vi "ROI 2 Trap Cluster.vi"(5 "Amplitudes":dbl[](array[numeric]), 6 "Switch X/Y":bool, 7 "Group":bool[](array[boolean]), 8 "Trap Cluster in":T2, 9 "Z":dbl[](array[numeric]), 10 "ROI":T1) -> (0 "Group out":bool[](array[boolean]), 1 "Z out":dbl[](array[numeric]), 2 "Amplitudes out":dbl[](array[numeric]), 3 "Trap Cluster Out":T2, 4 "Update display":bool)   [LabVIEW 8.6]
uses:
  Trap cluster.ctl
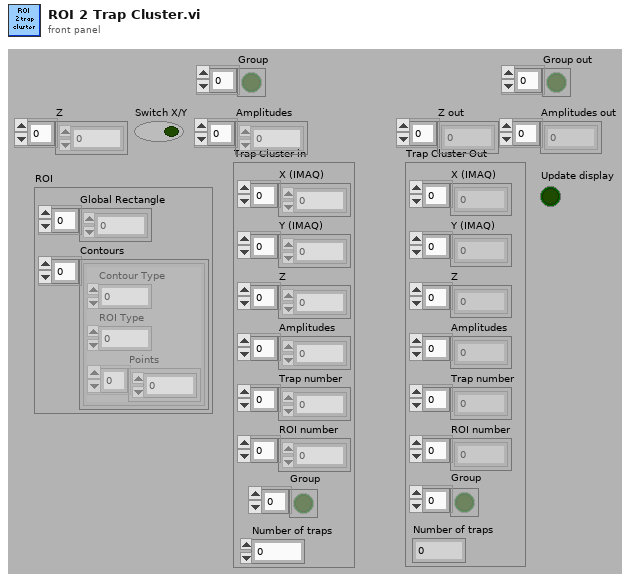
[diagram p1: front panel]
types:
  T1 = cluster{"Global Rectangle":i32[], "Contours":cluster{"Contour Type":u32, "ROI Type":u32, "Points":i32[]}[]}
  T2 = typedef "Trap cluster.ctl" = cluster{"X (IMAQ)":dbl[], "Y (IMAQ)":dbl[], "Z":dbl[], "Amplitudes":dbl[], "Trap number":i32[], "ROI number":i32[], "Number of traps":i32, "Group":bool[]}
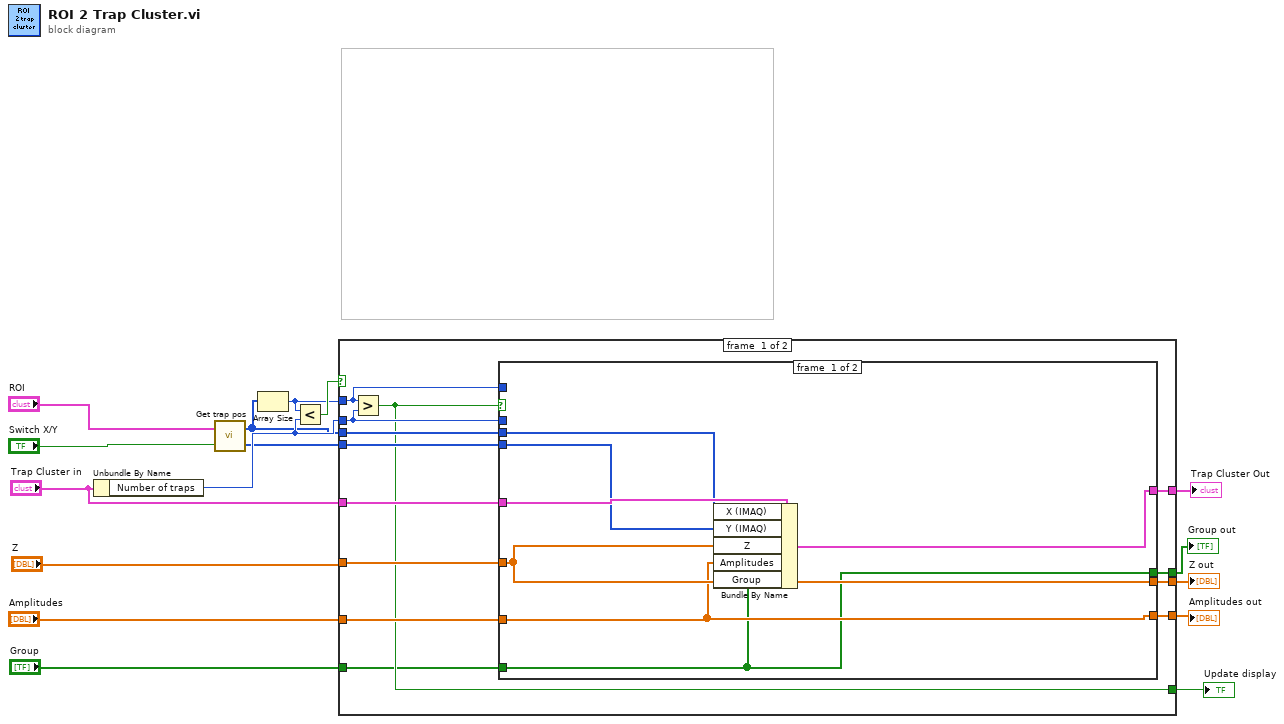
[diagram p0: block diagram]
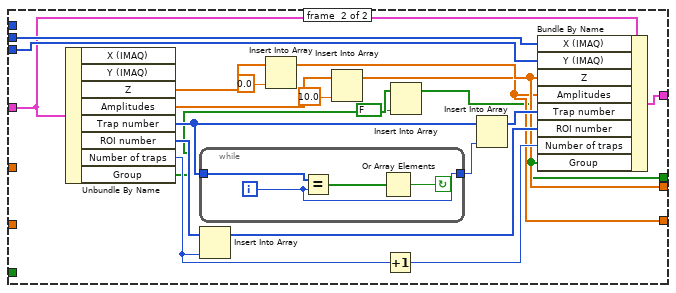
[diagram p2: hidden frame]
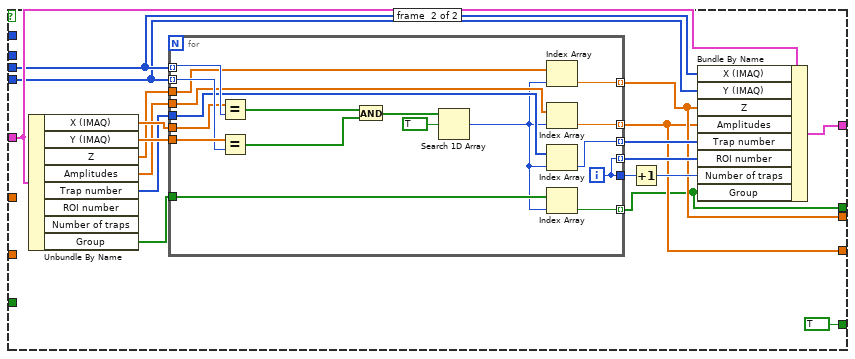
[diagram p3: hidden frame]
diagram:
  n1 = Unbundle By Name("Trap Cluster in") -> ("Number of traps"=w16:i32)
  n2 = call "Get trap pos.vi"("Switch X/Y"="Switch X/Y", "ROI"="ROI") -> ("Trap positions Y (IMAQ coordinates)"=w12:i32[], "Trap positions X (IMAQ coordinates)"=w11:i32[])
  n3 = Array Size(array=w11) -> (size(s)=w9:i32)
  n4 = Less?(x=w9, y=w16) -> (x < y?=w10:bool)
  n5 = case shown="False" w10 {
    tunnel: w12 -> [w28 w74]
    tunnel: w11 -> [w29 w75]
    tunnel: w9 -> [w24 _]
    tunnel: w16 -> [w27 _]
    tunnel: "Trap Cluster in" -> [w26 w76]
    tunnel: [w25 w66] -> w15
    tunnel: "Z" -> [w23 _]
    tunnel: [w22 w65] -> w6
    tunnel: [w21 w64] -> w5
    tunnel: "Amplitudes" -> [w20 _]
    tunnel: [w19 TRUE] -> w3
    tunnel: [w17 w61] -> w2
    tunnel: "Group" -> [w18 _]
    frame #0 {
      n6 = Greater?(x=w24, y=w27) -> (0:w19:bool)
      n7 = case shown="True" w19 {
        tunnel: [w33 w42] -> w25
        tunnel: w29 -> [w35 w56]
        tunnel: w28 -> [w34 w55]
        tunnel: w27 -> [_ _]
        tunnel: w26 -> [w36 w54]
        tunnel: w24 -> [_ _]
        tunnel: w23 -> [w32 _]
        tunnel: [w32 w41] -> w22
        tunnel: [w31 w40] -> w21
        tunnel: w20 -> [w31 _]
        tunnel: w18 -> [w30 _]
        tunnel: [w30 w37] -> w17
        frame #0 {
          n8 = Bundle By Name(cluster=w36, "X (IMAQ)"=w35, "Y (IMAQ)"=w34, "Z"=w32, "Amplitudes"=w31, "Group"=w30) -> (w33:T2)
        }
        frame #1 {
          n9 = Unbundle By Name(w54) -> ("Z"=w51:dbl[], "Amplitudes"=w49:dbl[], "Trap number"=w53:i32[], "ROI number"=w45:i32[], "Number of traps"=w44:i32, "Group"=w39:bool[])  [unwired: 2 out]
          n10 = while {
            tunnel: w53 -> [w60]
            tunnel: [w57] -> w46
            i -> [w57]
            stop <- w58 continue-if-true
            n11 = Equal?(x=w60, y=w57) -> (x = y?=w59:bool[])
            n12 = Or Array Elements(Boolean array=w59) -> (logical OR=w58:bool)
          }
          n13 = Insert Into Array(array=w45, new element=w44) -> (w43:i32[])  [unwired: 1 in]
          n14 = Insert Into Array(array=w51, new element=sgl 0.0 ("new element/subarray")) -> (w41:dbl[])  [unwired: 1 in]
          n15 = Insert Into Array(array=w49, new element=sgl 10.0 ("new element/subarray")) -> (w40:dbl[])  [unwired: 1 in]
          n16 = Increment(x=w44) -> (x+1=w47:i32)
          n17 = Insert Into Array(array=w39, new element=FALSE ("new element/subarray")) -> (w37:bool[])  [unwired: 1 in]
          n18 = Insert Into Array(array=w53, new element=w46) -> (w52:i32[])  [unwired: 1 in]
          n19 = Bundle By Name(cluster=w54, "X (IMAQ)"=w56, "Y (IMAQ)"=w55, "Z"=w41, "Amplitudes"=w40, "Trap number"=w52, "ROI number"=w43, "Number of traps"=w47, "Group"=w37) -> (w42:T2)
        }
      }
    }
    frame #1 {
      n20 = Unbundle By Name(w76) -> ("X (IMAQ)"=w78:dbl[], "Y (IMAQ)"=w77:dbl[], "Z"=w73:dbl[], "Amplitudes"=w72:dbl[], "Trap number"=w71:i32[], "Group"=w62:bool[])  [unwired: 2 out]
      n21 = for {
        tunnel: w78 -> [w93]
        tunnel: w75 -> [w96] mode=indexing
        tunnel: w77 -> [w95]
        tunnel: w74 -> [w94] mode=indexing
        tunnel: w73 -> [w90]
        tunnel: w72 -> [w89]
        tunnel: w71 -> [w88]
        tunnel: [w87] -> w65 mode=indexing
        tunnel: [w86] -> w64 mode=indexing
        tunnel: [w85] -> w70 mode=indexing
        tunnel: [w84] -> w69 mode=indexing
        tunnel: [w84] -> w68
        tunnel: w62 -> [w81]
        tunnel: [w79] -> w61 mode=indexing
        i -> [w84]
        n22 = Equal?(x=w93, y=w96) -> (x = y?=w92:bool[])
        n23 = Equal?(x=w95, y=w94) -> (x = y?=w91:bool[])
        n24 = And(x=w92, y=w91) -> (x .and. y?=w83:bool[])
        n25 = Search 1D Array(1D array=w83, element=TRUE) -> (index of element=w80:i32)  [unwired: 1 in]
        n26 = Index Array(array=w90, index=w80) -> (element=w87:dbl)
        n27 = Index Array(array=w89, index=w80) -> (element=w86:dbl)
        n28 = Index Array(array=w88, index=w80) -> (element=w85:i32)
        n29 = Index Array(array=w81, index=w80) -> (element=w79:bool)
      }
      n30 = Increment(x=w68) -> (x+1=w67:i32)
      n31 = Bundle By Name(cluster=w76, "X (IMAQ)"=w75, "Y (IMAQ)"=w74, "Z"=w65, "Amplitudes"=w64, "Trap number"=w70, "ROI number"=w69, "Number of traps"=w67, "Group"=w61) -> (w66:T2)
    }
  }
  "Trap Cluster Out" <- w15
  "Z out" <- w6
  "Amplitudes out" <- w5
  "Update display" <- w3
  "Group out" <- w2
